vi "Main_Taper.vi"() -> ()   [LabVIEW 2014]
uses:
  <vilib>/Instr/_visa.llb/VISA Configure Serial Port (Instr).vi
panel:
  in  "Tab Control":enum32{"COM Config", "Taper", "Manual"}(tab)=enum."Taper"
  in  "Stop Taper":bool
  out "COM_OK":bool
  in  "Send":bool
  in  "Start":bool
  in  "COM Write":string="AA;\nVL15.0000;\nAX;\nLS4;\nMR4.0000;\nGO;\nMR-4.0000;\nGO;\nLE;\nAA;\nVL1.0000,0.2000,0.2000;\nMR,-5.7085,-5.7085;\nGO;\nAX;\nLS4.0000;\nMR4.0000;\nGO;\nMR-4.0000\nGO;\nLE;"
  in  "COM Config":T1={"VISA resource name"="COM4", "baud rate"=9600, "data bits"=8, "parity"=enum."None", "stop bits"=10, "flow control"=0} {"flow control" items=["None"=0, "XON/XOFF"=1, "RTS/CTS"=2, "DTR/DSR"=4]; "data bits" min=5 max=8 step=1}
  in  "Stop Button":bool
  out "Taper Finish":bool
  in  "Diametro taper (um)":dbl=30.0
  in  "Longitud waist (mm)":dbl=8.0
  in  "VELOCIDAD  STRETCHING":dbl=0.2
  in  "VELOCIDAD QUEMADOR (mm/s)":dbl=1.0
  out "TIEMPO REQUERIDO   (s)":dbl=30.67566044613625
  in  "Diametro inicial(um)":dbl=125.0
  in  "Calcular movimiento":bool
  out "Estiramiento (mm)":dbl=-11.416930845121167
  in  "Oscilaciones Precalentamiento":u8=4
  in  "Velocidad Precalentamiento":dbl=10.0
  in  "Velocidad Z":dbl=2.0
  in  "Velocidad Y":dbl=2.0
  in  "Velocidad X":dbl=2.0
  in  "Move Z (mm)":dbl=10.0
  in  "Move Y (mm)":dbl=10.0
  in  "Move X (mm)":dbl
  in  "Escribir Valores":bool
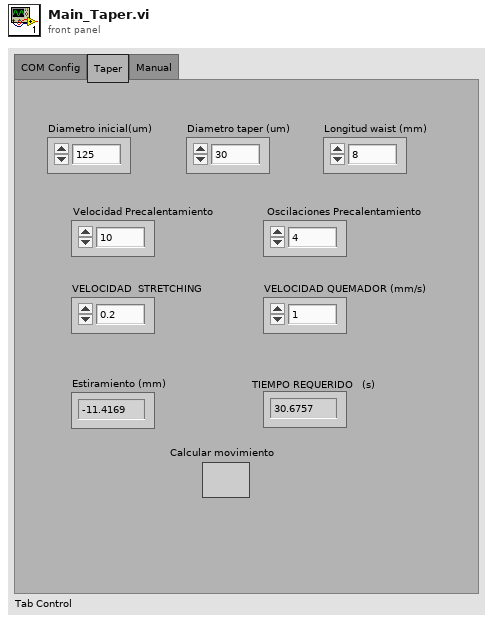
[diagram p1: front panel]
types:
  T1 = cluster{"VISA resource name":refnum<visa-resource-name>, "baud rate":u32, "data bits":u16, "parity":enum16{"None", "Odd", "Even", "Mark", "Space"}, "stop bits":u16, "flow control":u16}
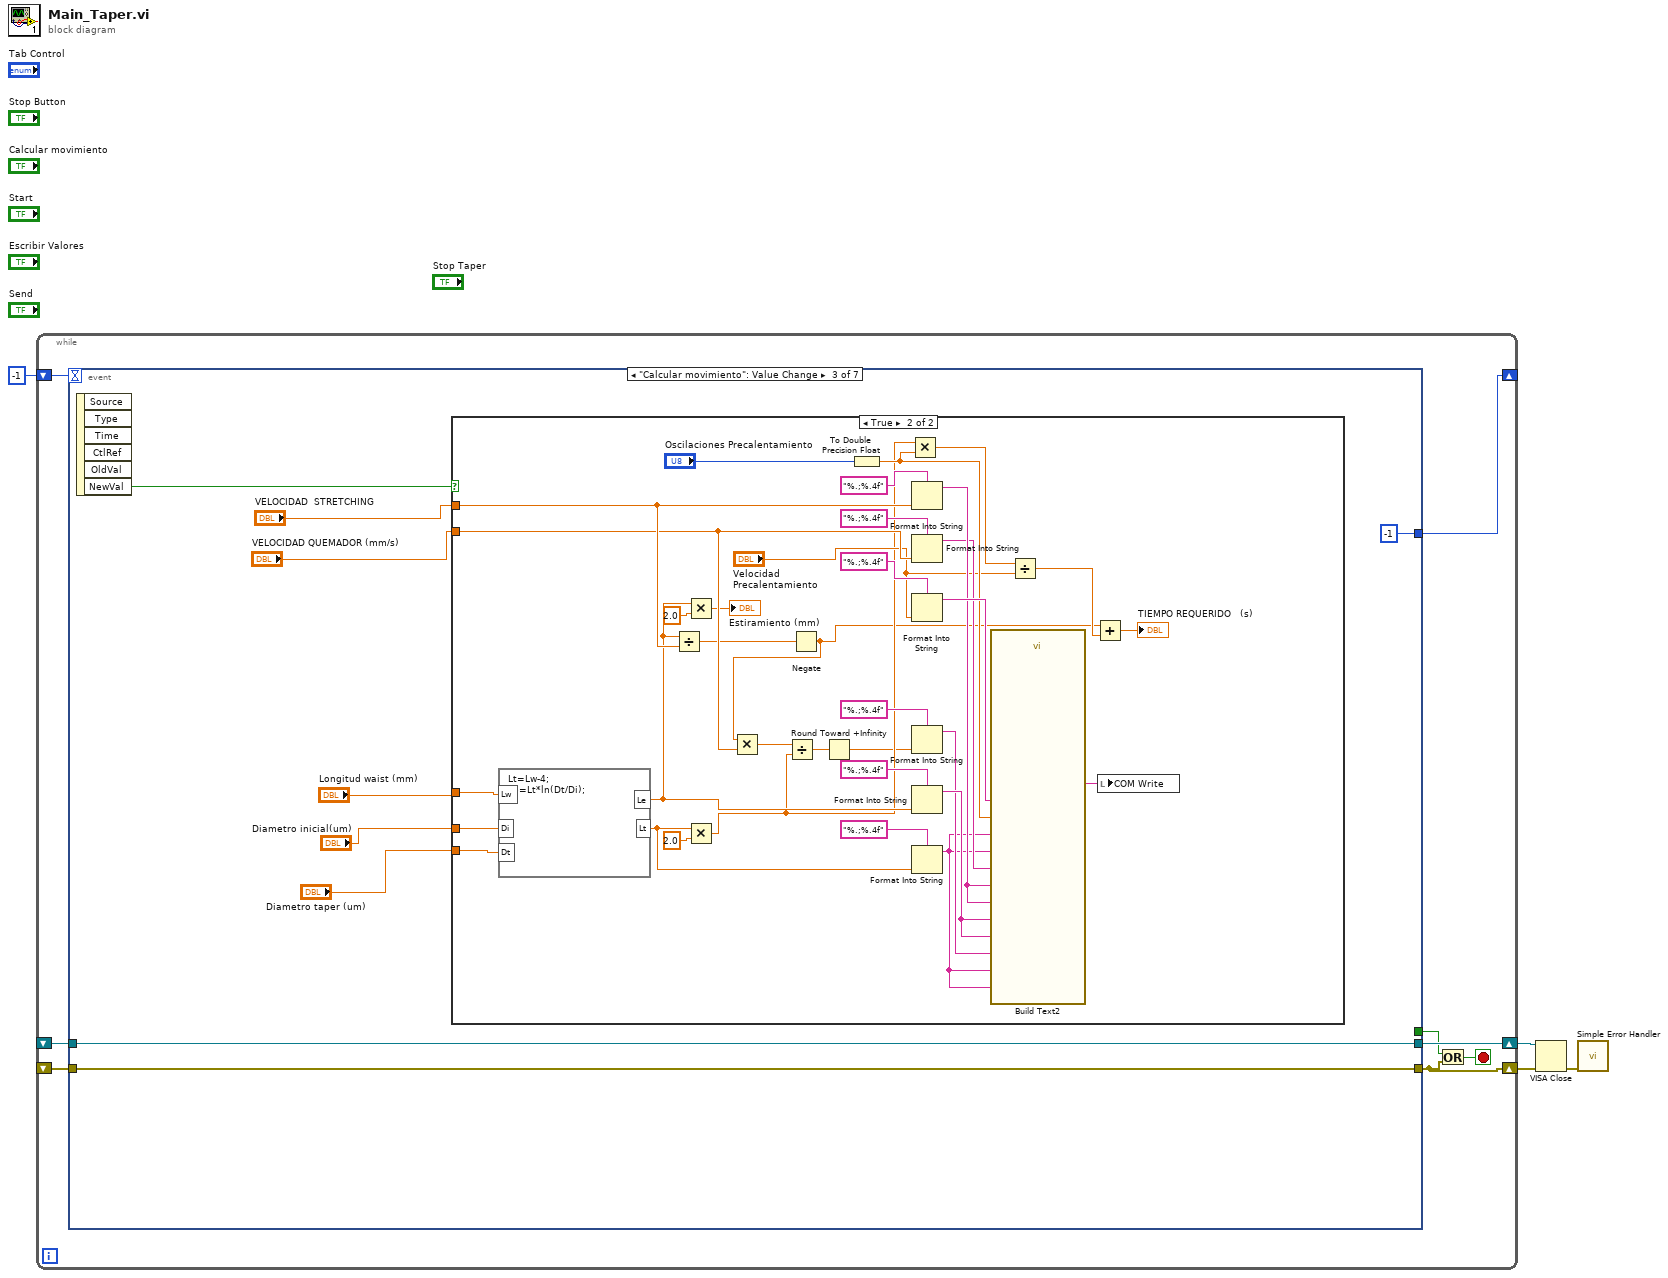
[diagram p0: block diagram]
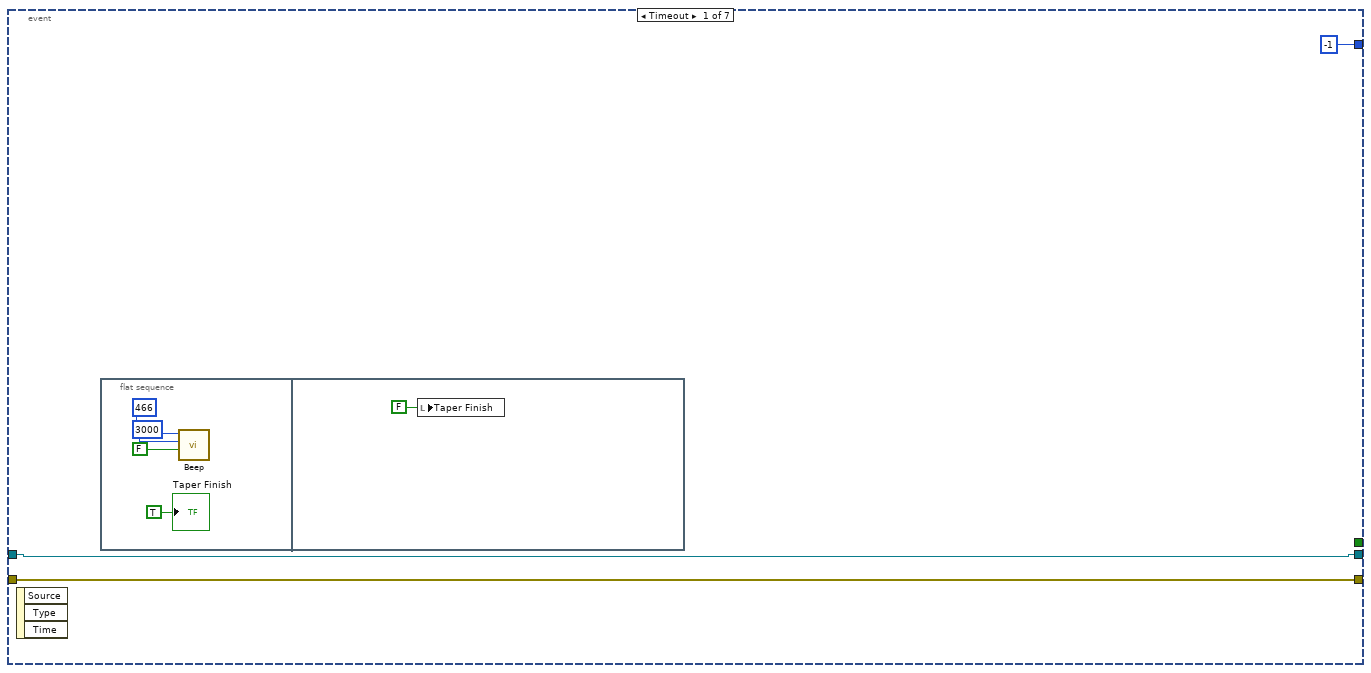
[diagram p2: hidden frame]
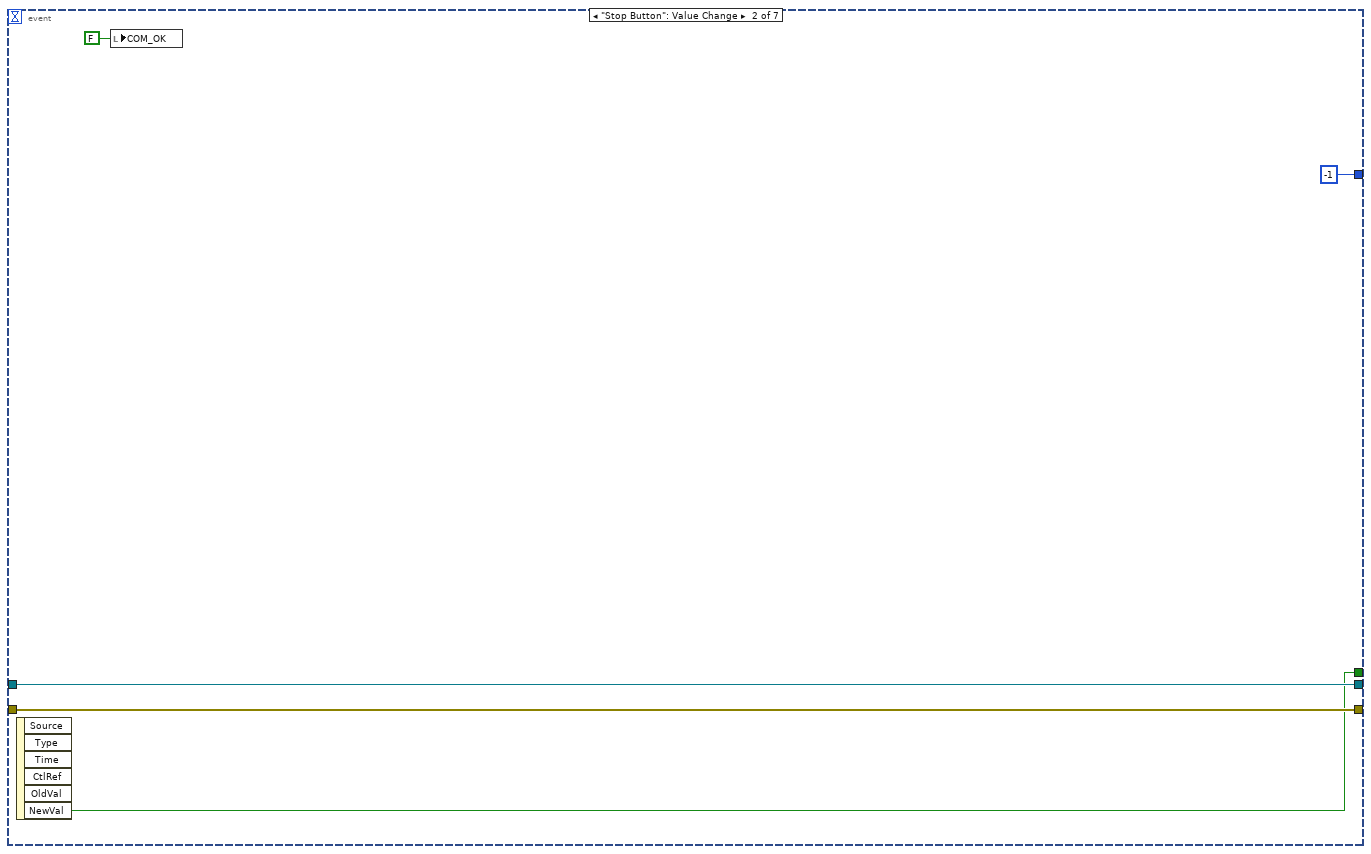
[diagram p3: hidden frame]
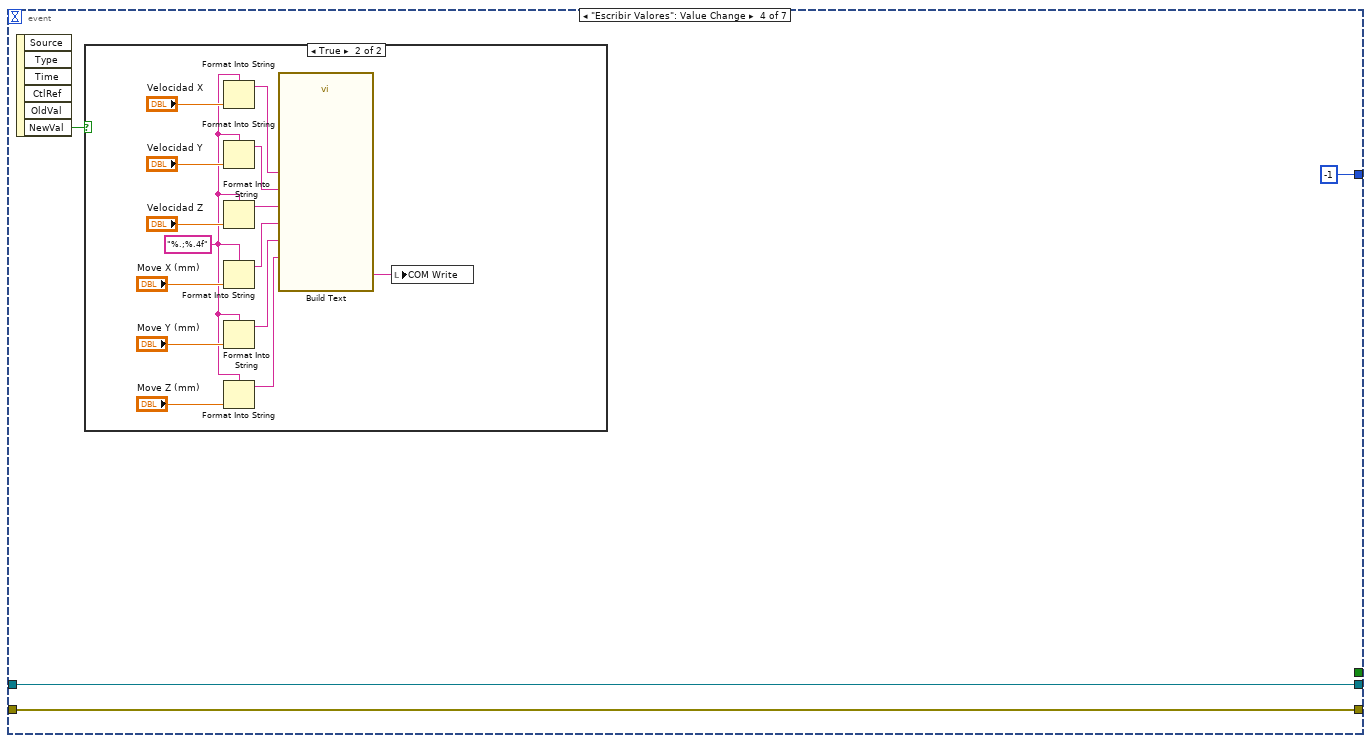
[diagram p5: hidden frame]
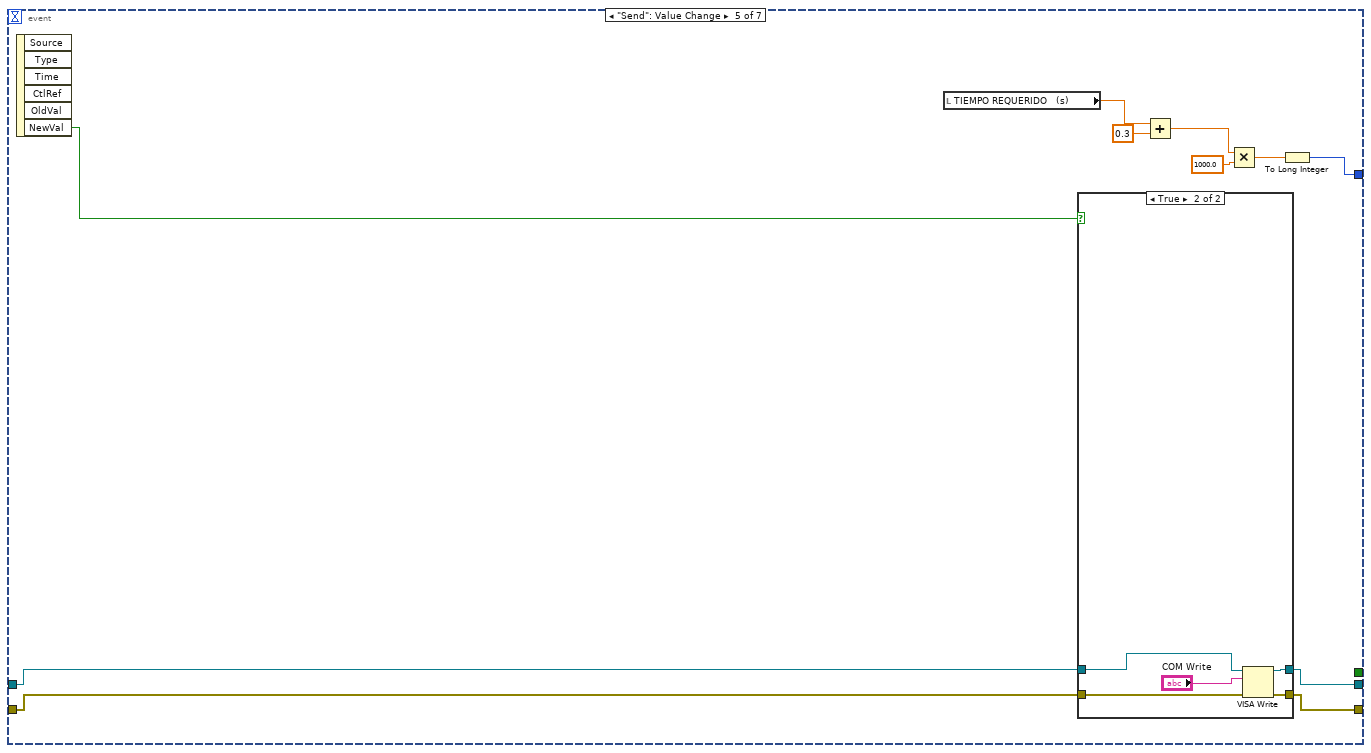
[diagram p7: hidden frame]
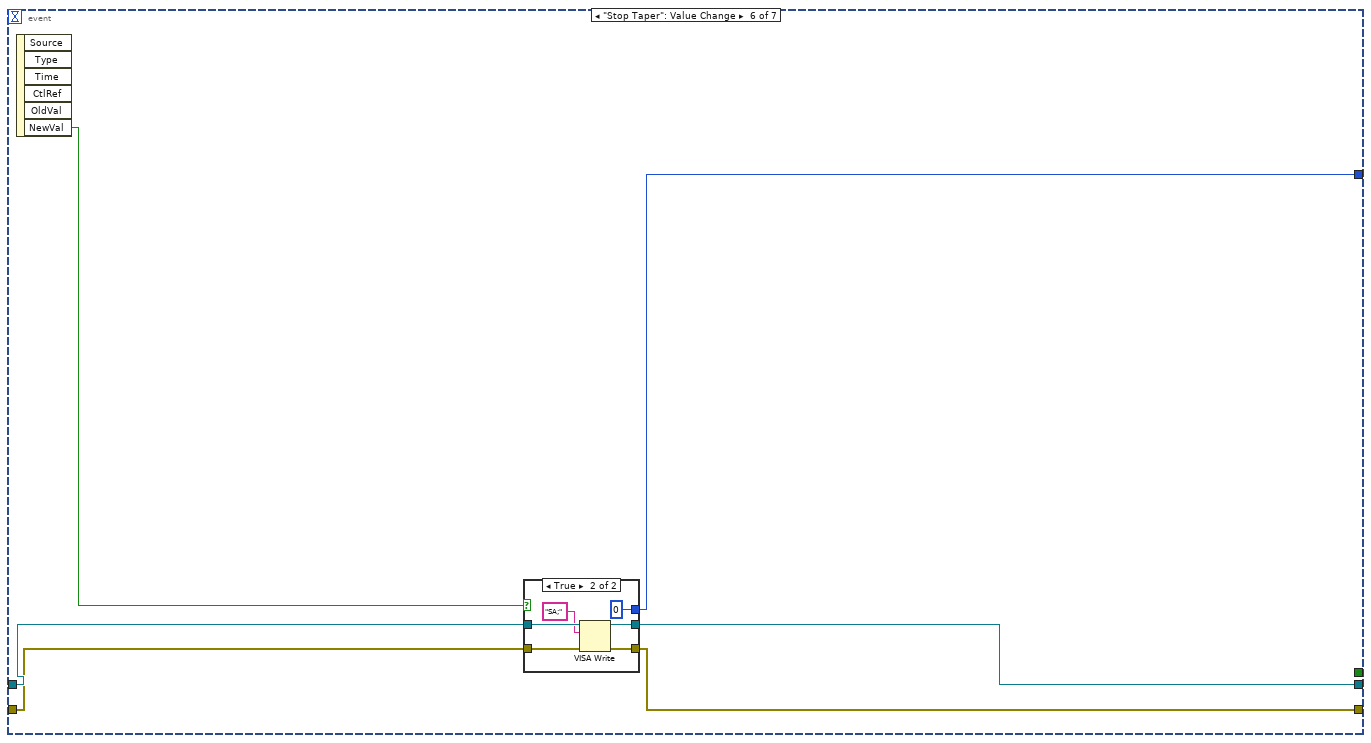
[diagram p9: hidden frame]
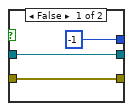
[diagram p10: hidden frame]
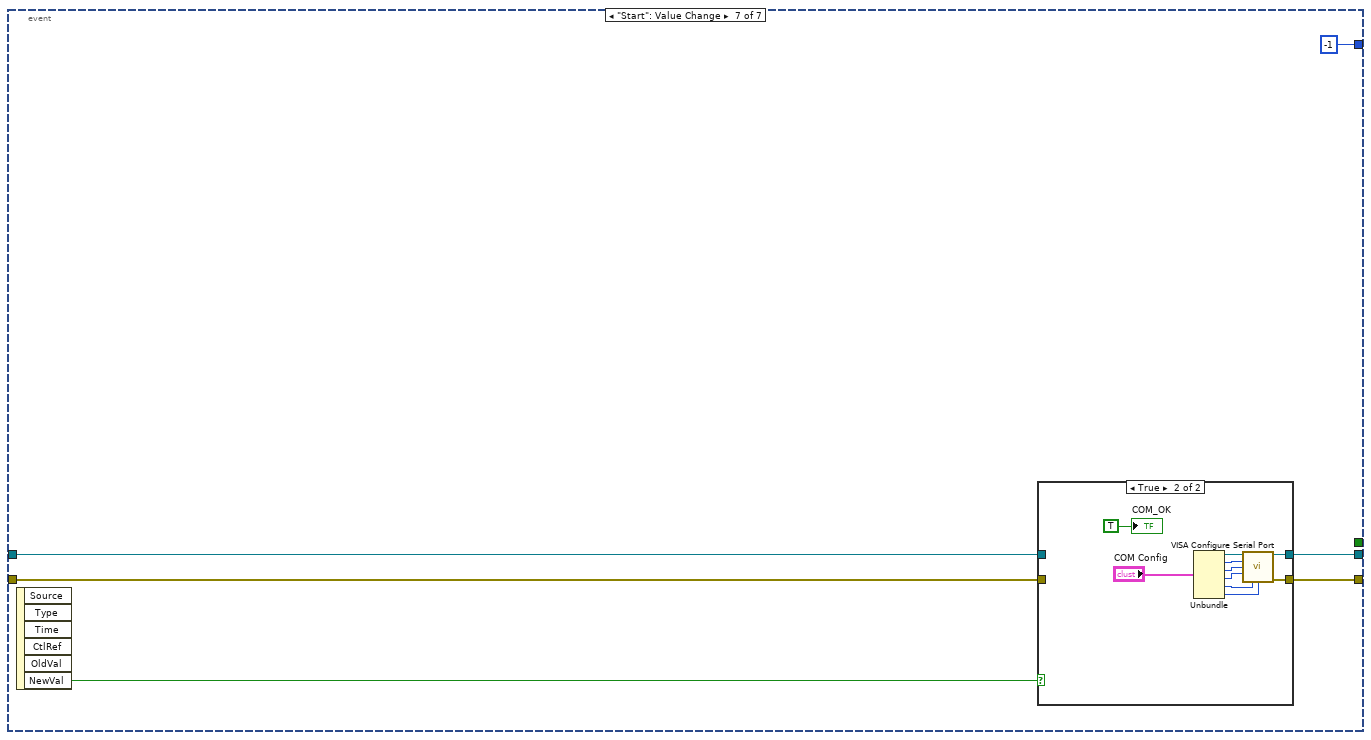
[diagram p11: hidden frame]
diagram:
  n1 = while {
    shift-right: [w10] -> w4
    shift-left: _ -> [w12]
    shift-right: [w7] -> w3
    shift-left: _ -> [w11]
    shift-right: [w5] -> _
    shift-left: -1 -> [w6]
    stop <- w8 stop-if-true
    n2 = event shown="[2] \"Calcular movimiento\": Value Change" {
      selector: _ -> [_ _ _ _ _ _ _]
      dyn-events: _ -> [_ _ _ _ _ _ _]
      timeout: w6 -> [_ _ _ _ _ _ _]
      tunnel: [w15 w25 w28 w72 w95 w108 w125] -> w10
      tunnel: [w14 w24 w27 w71 w94 w107 w124] -> w7
      tunnel: w12 -> [w15 w25 w28 w72 w97 w110 w123]
      tunnel: w11 -> [w14 w24 w27 w71 w96 w109 w122]
      tunnel: [_ w23 _ _ _ _ _] -> w9
      tunnel: [-1 -1 -1 -1 w91 w106 -1] -> w5
      event Timeout {
        n3 = event-data() -> ()  [unwired: 1 in, 3 out]
        n4 = flat-sequence {
          frame #0 {
            n5 = call <vilib>:"Beep.vi"("use system alert? (T)"=FALSE, "duration (msec)"=u32 3000, "frequency (Hz)"=u32 466) -> ()  [unwired: 9 in]
            "Taper Finish" <- TRUE ("Taper FInish")
          }
          frame #1 {
            n6 = local write "Taper Finish"(FALSE ("Taper FInish")) -> ()
          }
        }
      }
      event "Stop Button": Value Change {
        n7 = event-data() -> ("NewVal"=w23:bool)  [unwired: 1 in, 5 out]
        n8 = local write "COM_OK"(FALSE ("COM_OK")) -> ()
      }
      event "Calcular movimiento": Value Change {
        n9 = event-data() -> ("NewVal"=w29:bool)  [unwired: 1 in, 5 out]
        n10 = case shown="True" w29 {
          tunnel: "VELOCIDAD  STRETCHING" -> [_ w58]
          tunnel: "Diametro inicial(um)" -> [_ w69]
          tunnel: "Diametro taper (um)" -> [_ w68]
          tunnel: "Longitud waist (mm)" -> [_ w67]
          tunnel: "VELOCIDAD QUEMADOR (mm/s)" -> [_ w57]
          frame False {
          }
          frame True {
            n11 = formula code="Lt=Lw-4;\nLe=Lt*ln(Dt/Di);"("Lw"=w67, "Di"=w69, "Dt"=w68) -> ("Le"=w38:dbl, "Lt"=w47:dbl)
            n12 = Divide(x=w38, y=w58) -> (x/y=w41:dbl)
            n13 = Multiply(x=w38, y=2.0) -> (x*y=→"Estiramiento (mm)":dbl)
            n14 = Multiply(x=w47, y=2.0) -> (x*y=w37:dbl)
            n15 = Negate(x=w41) -> (-x=w36:dbl)
            n16 = Multiply(x=w36, y=w57) -> (x*y=w66:dbl)
            n17 = Divide(x=w66, y=w37) -> (x/y=w52:dbl)
            n18 = Round Toward +Infinity(x=w52) -> (ceil(x): smallest int >= x=w35:dbl)
            n19 = To Double Precision Float(number="Oscilaciones Precalentamiento") -> (double precision float=w43:dbl)
            n20 = Multiply(x=w37, y=w43) -> (x*y=w45:dbl)
            n21 = Format Into String(format string="%.;%.4f", w58) -> (resulting string=w56:string)  [unwired: 2 in, 1 out]
            n22 = Format Into String(format string="%.;%.4f", w57) -> (resulting string=w55:string)  [unwired: 2 in, 1 out]
            n23 = Format Into String(format string="%.;%.4f", "Velocidad Precalentamiento") -> (resulting string=w59:string)  [unwired: 2 in, 1 out]
            n24 = Format Into String(format string="%.;%.4f", w35) -> (resulting string=w51:string)  [unwired: 2 in, 1 out]
            n25 = Format Into String(format string="%.;%.4f", w38) -> (resulting string=w54:string)  [unwired: 2 in, 1 out]
            n26 = Format Into String(format string="%.;%.4f", w47) -> (resulting string=w50:string)  [unwired: 2 in, 1 out]
            n27 = call "Build Text2"("Velocidad Precalentamiento"=w59, "Oscilaciones Precalentamiento"=w43, "movimiento del quemador"=w50, "movimiento del quemador 1"=w50, "velocidad X"=w55, "velocidad Y"=w56, "velocidad Z"=w56, "movimiento Y"=w54, "movimiento Z"=w54, "numero de oscilaciones del quemador"=w51, "movimiento del quemador 2"=w50, "movimiento del quemador 3"=w50) -> ("Result"=w65:string)  [unwired: 14 in, 1 out]
            n28 = Divide(x=w45, y="Velocidad Precalentamiento") -> (x/y=w40:dbl)
            n29 = Add(x=w36, y=w40) -> (x+y=→"TIEMPO REQUERIDO   (s)":dbl)
            n30 = local write "COM Write"(w65) -> ()
          }
        }
      }
      event "Escribir Valores": Value Change {
        n31 = event-data() -> ("NewVal"=w73:bool)  [unwired: 1 in, 5 out]
        n32 = case shown="True" w73 {
          frame False {
          }
          frame True {
            w81 = "%.;%.4f" ("format string")
            n33 = Format Into String(format string=w81, "Velocidad X") -> (resulting string=w80:string)  [unwired: 2 in, 1 out]
            n34 = Format Into String(format string=w81, "Velocidad Y") -> (resulting string=w79:string)  [unwired: 2 in, 1 out]
            n35 = Format Into String(format string=w81, "Velocidad Z") -> (resulting string=w78:string)  [unwired: 2 in, 1 out]
            n36 = Format Into String(format string=w81, "Move X (mm)") -> (resulting string=w77:string)  [unwired: 2 in, 1 out]
            n37 = Format Into String(format string=w81, "Move Y (mm)") -> (resulting string=w76:string)  [unwired: 2 in, 1 out]
            n38 = Format Into String(format string=w81, "Move Z (mm)") -> (resulting string=w75:string)  [unwired: 2 in, 1 out]
            n39 = call "Build Text"("movimiento X"=w77, "movimiento Z"=w75, "velocidad X"=w80, "velocidad Y"=w79, "velocidad Z"=w78, "movimiento Y"=w76) -> ("Result"=w74:string)  [unwired: 8 in, 1 out]
            n40 = local write "COM Write"(w74) -> ()
          }
        }
      }
      event "Send": Value Change {
        n41 = event-data() -> ("NewVal"=w98:bool)  [unwired: 1 in, 5 out]
        n42 = local read "TIEMPO REQUERIDO   (s)"() -> (w90:dbl)
        n43 = case shown="True" w98 {
          tunnel: w96 -> [w100 w104]
          tunnel: w97 -> [w99 w105]
          tunnel: [w99 w102] -> w95
          tunnel: [w100 w101] -> w94
          frame False {
          }
          frame True {
            n44 = VISA Write(VISA resource name=w105, write buffer="COM Write", error in (no error)=w104) -> (VISA resource name out=w102:refnum<visa-resource-name>, error out=w101:errorcluster)  [unwired: 1 out]
          }
        }
        n45 = Add(x=w90, y=0.3) -> (x+y=w88:dbl)
        n46 = Multiply(x=w88, y=1000.0) -> (x*y=w92:dbl)
        n47 = To Long Integer(number=w92) -> (32bit integer=w91:i32)
      }
      event "Stop Taper": Value Change {
        n48 = event-data() -> ("NewVal"=w111:bool)  [unwired: 1 in, 5 out]
        n49 = case shown="True" w111 {
          tunnel: w110 -> [w114 w120]
          tunnel: w109 -> [w113 w119]
          tunnel: [w114 w118] -> w108
          tunnel: [w113 w117] -> w107
          tunnel: [-1 0] -> w106
          frame False {
          }
          frame True {
            n50 = VISA Write(VISA resource name=w120, write buffer="SA;", error in (no error)=w119) -> (VISA resource name out=w118:refnum<visa-resource-name>, error out=w117:errorcluster)  [unwired: 1 out]
          }
        }
      }
      event "Start": Value Change {
        n51 = event-data() -> ("NewVal"=w126:bool)  [unwired: 1 in, 5 out]
        n52 = case shown="True" w126 {
          tunnel: [w127 w131] -> w124
          tunnel: [w128 w130] -> w125
          tunnel: w123 -> [w128 _]
          tunnel: w122 -> [w127 _]
          frame False {
          }
          frame True {
            n53 = Unbundle("COM Config") -> ("VISA resource name"=w137:refnum<visa-resource-name>, "baud rate"=w136:u32, "data bits"=w135:u16, "parity"=w132:enum16{"None", "Odd", "Even", "Mark", "Space"}, "stop bits"=w134:u16, "flow control"=w133:u16)
            n54 = call-poly "VISA Configure Serial Port"("VISA resource name"=w137, "baud rate (9600)"=w136, "data bits (8)"=w135, "parity (0:none)"=w132, "stop bits (10: 1 bit)"=w134, "flow control (0:none)"=w133) -> ("VISA resource name out"=w130:refnum<visa-resource-name>, "error out"=w131:errorcluster)  [unwired: 8 in]
            "COM_OK" <- TRUE ("COM_OK")
          }
        }
      }
    }
    n55 = Or(x=w9, y=w7) -> (x .or. y?=w8:bool)
  }
  n56 = VISA Close(VISA resource name=w4, error in (no error)=w3) -> (error out=w2:errorcluster)
  n57 = call <vilib>:"Simple Error Handler.vi"("error in (no error)"=w2) -> ()  [unwired: 4 in, 5 out]
